vi "Init.vi"(3 "Container State":T3, 4 "Previous State":variant, 5 "Previous Version":T2) -> (2 "Current State":T1)   [LabVIEW 2015, in "Tone (G3).xctl"]
uses:
  Tone (G3).xctl
  State.ctl
  Utility VIs/Controls/KNumeric (DBL)/KNumeric (DBL).xctl
  Utility VIs/Controls/KCheckbox/KCheckbox.xctl
  <vilib>/_xctls/Container State.ctl
  <vilib>/_xctls/Version.ctl
  <vilib>/_xctls/XControlSupport.lvlib
panel:
  in  "Default Indicator State":T1={"enable menu"=TRUE, "ctls"={"Freq"=refnum, "Phase"=refnum, "Random"=refnum}}
  in  "Default Control State":T1={"enable menu"=TRUE, "ctls"={"Freq"=refnum, "Phase"=refnum, "Random"=refnum}}
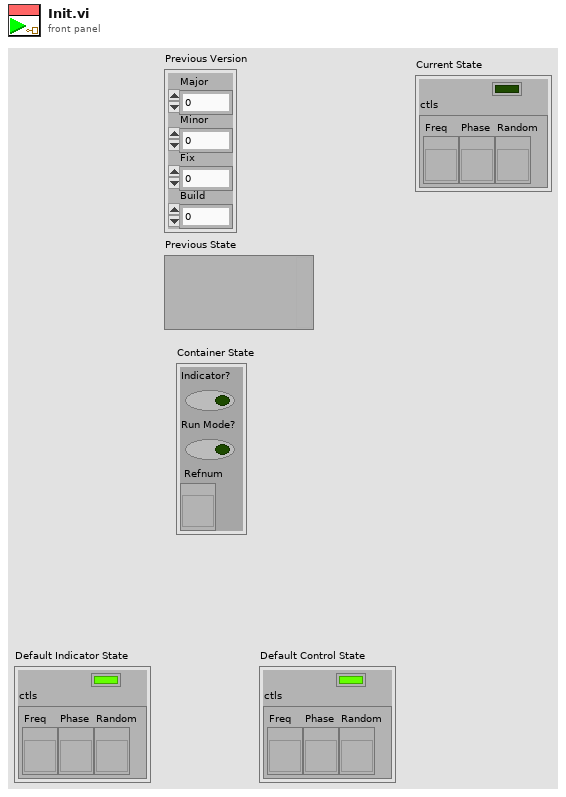
[diagram p1: front panel]
types:
  T1 = typedef "Tone (G3).xctl/State.ctl" = cluster{"enable menu":bool, "ctls":cluster{"Freq":refnum<vi>, "Phase":refnum<vi>, "Random":refnum<vi>}}
  T2 = typedef "XControlSupport.lvlib/Version.ctl" = cluster{"Major":u16, "Minor":u16, "Fix":u16, "Build":u16}
  T3 = typedef "XControlSupport.lvlib/Container State.ctl" = cluster{"Indicator?":bool, "Run Mode?":bool, " Refnum":refnum<vi>}
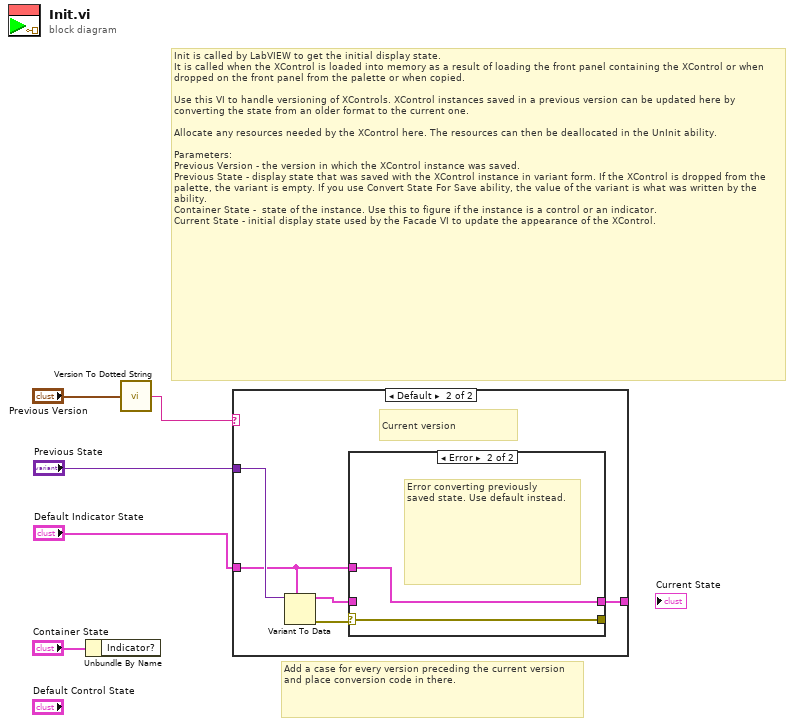
[diagram p0: block diagram]
diagram:
  # "Add a case for every version preceding the current version and place conversion code in there."
  # "Init is called by LabVIEW to get the initial display state.\nIt is called when the XControl is loaded into memory as a result of loading the front panel containing the XControl or when dropped on the front panel from the palette or when copied.\n\nUse this VI to handle versioning of XControls. XControl instances saved in a previous version can be updated here by converting the state from an older format to the current one.\n\nAllocate any resources needed by the XControl here. The resources can then be deallocated in the UnInit ability.\n\nParameters:\nPrevious Version - the version in which the XControl instance was saved.\nPrevious State - display state that was saved with the XControl instance in variant form. If the XControl is dropped from the palette, the variant is empty. If you use Convert State For Save ability, the value of the variant is what was written by the ability. \nContainer State -  state of the instance. Use this to figure if the instance is a control or an indicator.\nCurrent State - initial display state used by the Facade VI to update the appearance of the XControl."
  n1 = Unbundle By Name("Container State") -> ()  [unwired: 1 out]
  n2 = call <vilib>:"Version To Dotted String.vi"("Version"="Previous Version") -> ("String Version"=w2:string)
  n3 = case shown="Default" w2 {
    tunnel: "Previous State" -> [_ w11]
    tunnel: [w6 w7] -> _
    tunnel: "Default Indicator State" -> [w6 w8]
    frame "0.0.0.0" {
      # "Just created, use default state"
    }
    frame Default {
      # "Current version"
      n4 = Variant To Data(type=w8, Variant=w11) -> (data=w9:T1, error out=w10:errorcluster)  [unwired: 1 in]
      n5 = case shown="Error" w10 {
        selector: w10 -> [w13 w14]
        tunnel: w9 -> [w12 _]
        tunnel: [w12 w15] -> w7
        tunnel: w8 -> [_ w15]
        tunnel: [w13 w14] -> _
        frame No Error {
        }
        frame Error {
          # "Error converting previously \nsaved state. Use default instead."
        }
      }
    }
  }
